vi "SubVI Translate.vi"(8 "error in (no error)":errorcluster, 10 "reentrant VIs":string[](array[string]), 11 "SubVI in":refnum<vi>) -> (0 "error out":errorcluster, 1 "reentrant VIs out":string[](array[string]), 2 "transcripted code":string, 3 "transcriptor cluster":T1)   [LabVIEW 2014]
uses:
  types/LabVIEW Universal Transcriptor Cluster.ctl
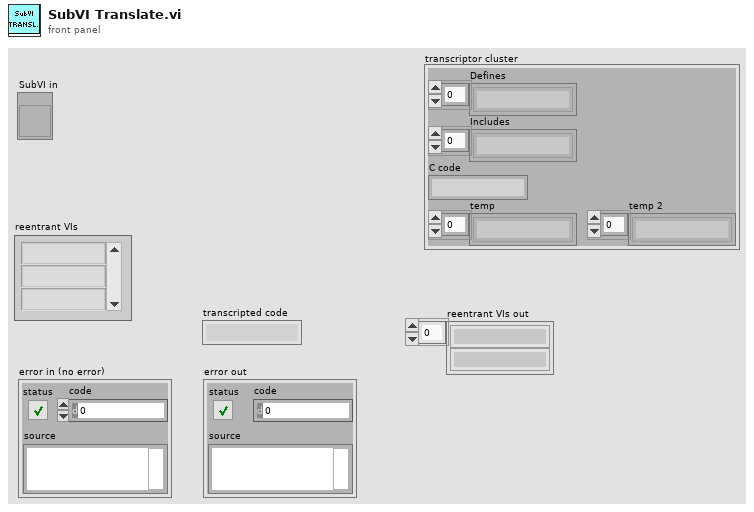
[diagram p1: front panel]
types:
  T1 = typedef "LabVIEW Universal Transcriptor Cluster.ctl" = cluster{"Defines":string[], "Includes":string[], "C code":string, "temp":string[], "temp 2":string[]}
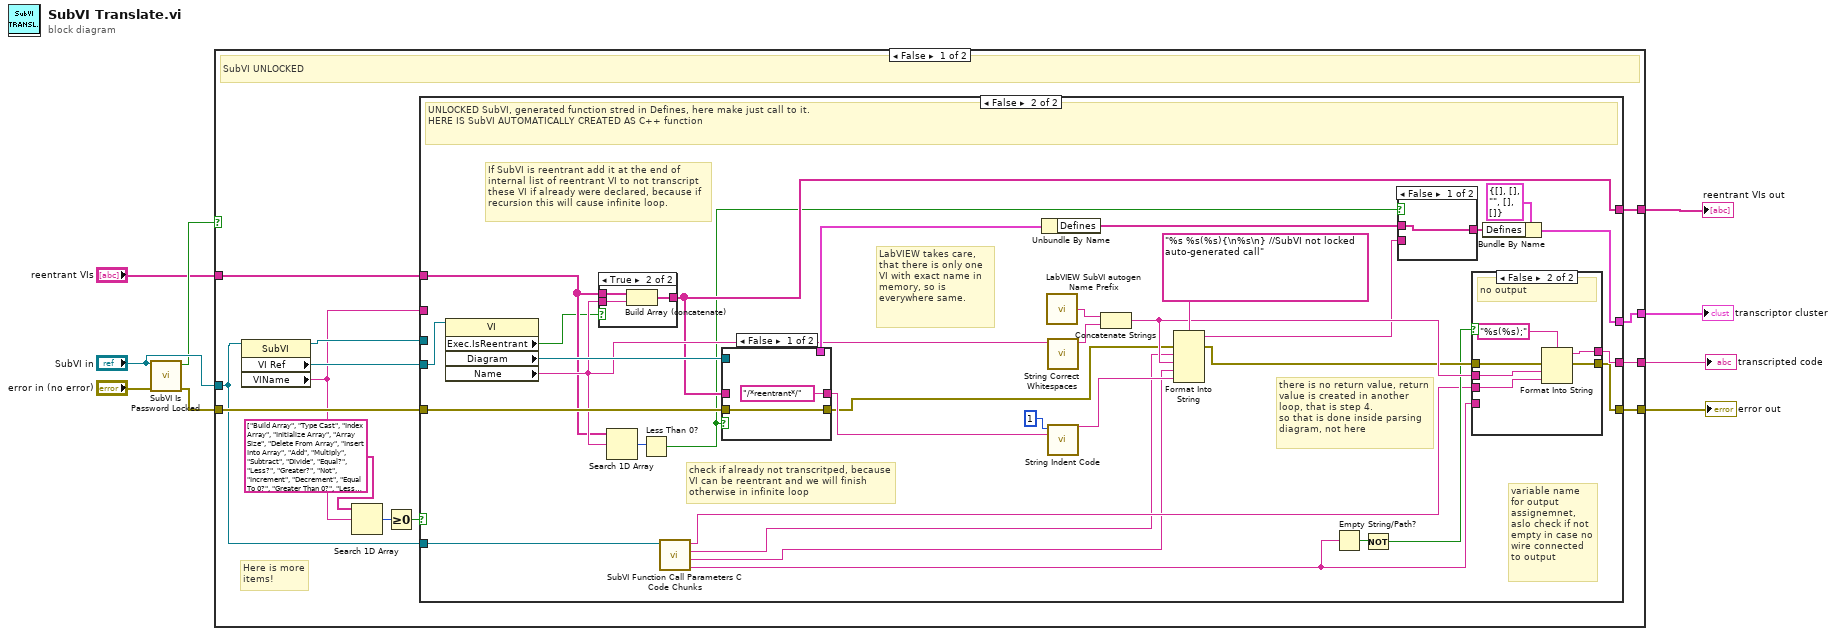
[diagram p0: block diagram]
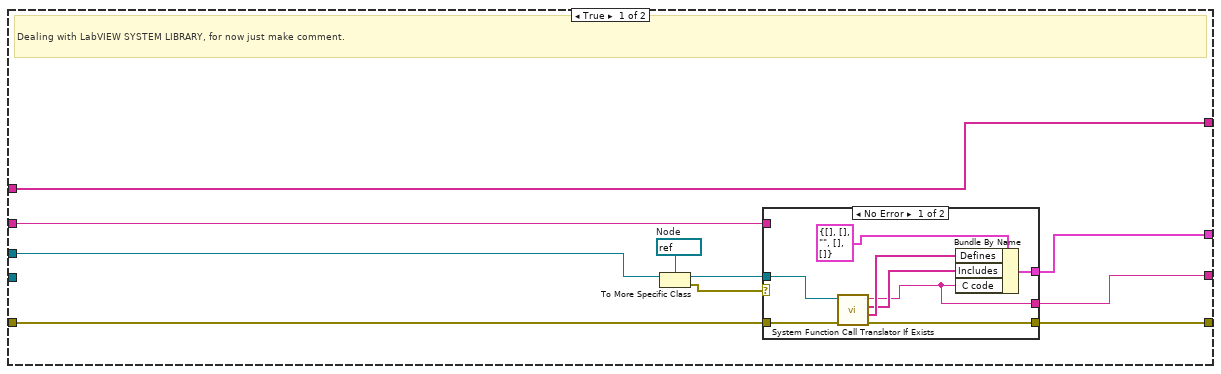
[diagram p2: hidden frame]
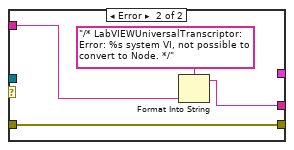
[diagram p3: hidden frame]
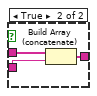
[diagram p4: hidden frame]
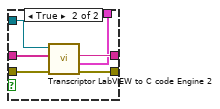
[diagram p6: hidden frame]
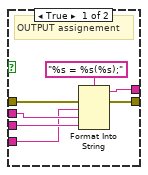
[diagram p7: hidden frame]
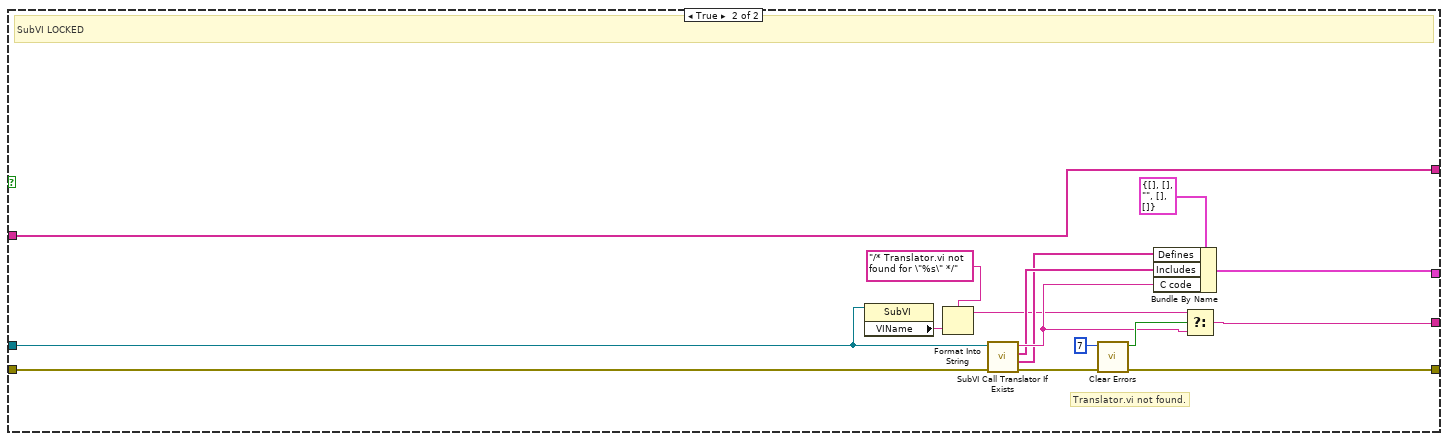
[diagram p8: hidden frame]
diagram:
  n1 = call "SubVI Is Password Locked.vi"("Error In"="error in (no error)", "SubVI ref"="SubVI in") -> ("Error Out"=w8:errorcluster, "isPasswordLocked?"=w5:bool)  [unwired: 8 in]
  n2 = case shown="False" w5 {
    tunnel: "SubVI in" -> [w12 w118]
    tunnel: [w20 w122] -> w7
    tunnel: w8 -> [w22 w121]
    tunnel: [w19 w120] -> w9
    tunnel: [w18 w119] -> w4
    tunnel: "reentrant VIs" -> [w11 w107]
    tunnel: [w10 w107] -> w1
    frame False {
      # "Here is more items!"
      # "SubVI UNLOCKED"
      n3 = property class="SubVI"(reference=w12) -> (reference out=w17:refnum<vi>, "VI Ref"=w21:refnum<vi>, "VIName"=w13:string)  [unwired: 1 in, 1 out]
      n4 = Search 1D Array(1D array=string[] ["Build Array", "Type Cast", "Index Array", "Initialize Array", "Array Size", "Delete From Array", "Insert Into Array", "Add", "Multiply", "Subtract", "Divide", "Equal?", "Less?", "Greater?", "Not", "Increment", "Decrement", "Equal To 0?", "Greater Than 0?", "Less Than 0?", "Greater Or Equal To 0?", "Greater Or Equal?", "Less Or Equal?", "Not Equal?", "Not Equal To 0?", "And", "Or", "Exclusive Or", "To Lower Case", "To Upper Case", "String Length", "String Subset", "Match Pattern", "Decimal String To Number", "Number To Fractional String", "Fract/Exp String To Number", "Number To Decimal String"], element=w13) -> (index of element=w16:i32)  [unwired: 1 in]
      n5 = Greater Or Equal To 0?(x=w16) -> (x >= 0?=w15:bool)
      n6 = case shown="False" w15 {
        tunnel: w22 -> [w30 w52]
        tunnel: w21 -> [_ w64]
        tunnel: [w32 w76] -> w20
        tunnel: [w29 w66] -> w19
        tunnel: w13 -> [w31 _]
        tunnel: [w27 w77] -> w18
        tunnel: w12 -> [_ w62]
        tunnel: w17 -> [w28 _]
        tunnel: w11 -> [w23 w48]
        tunnel: [w23 w47] -> w10
        frame True {
          w26 = refnum<vi> refnum  # Node
          # "Dealing with LabVIEW SYSTEM LIBRARY, for now just make comment."
          n7 = To More Specific Class(target class=w26, reference=w28) -> (specific class reference=w25:refnum<vi>, error out=w24:errorcluster)  [unwired: 1 in]
          n8 = case shown="No Error" w24 {
            tunnel: [w40 w44] -> w29
            tunnel: w25 -> [w39 _]
            tunnel: [w36 _] -> w27
            tunnel: [w35 w41] -> w32
            tunnel: w30 -> [w34 w44]
            tunnel: w31 -> [_ w42]
            frame No Error {
              n9 = call "System Function Call Translator If Exists.vi"("Error In"=w34, "Node Refnum"=w39) -> ("Error Out"=w40:errorcluster, "Defines"=w38:string[], "Includes"=w37:string[], "Replaced Code"=w35:string)  [unwired: 6 in]
              n10 = Bundle By Name(cluster=T1 {"Defines"=[], "Includes"=[], "C code"="", "temp"=[], "temp 2"=[]} ("input cluster"), "Defines"=w38, "Includes"=w37, "C code"=w35) -> (w36:T1)
            }
            frame Error {
              n11 = Format Into String(format string="/* LabVIEWUniversalTranscriptor: Error: %s system VI, not possible to convert to Node. */" ("Replaced Code"), w42) -> (resulting string=w41:string)  [unwired: 2 in, 1 out]
            }
          }
        }
        frame False {
          # "If SubVI is reentrant add it at the end of internal list of reentrant VI to not transcript these VI if already were declared, because if recursion this will cause infinite loop."
          # "check if already not transcritped, because VI can be reentrant and we will finish otherwise in infinite loop"
          # "variable name for output assignemnet, aslo check if not empty in case no wire connected to output"
          # "there is no return value, return value is created in another loop, that is step 4.\nso that is done inside parsing diagram, not here"
          # "LabVIEW takes care, that there is only one VI with exact name in memory, so is everywhere same."
          # "UNLOCKED SubVI, generated function stred in Defines, here make just call to it.\nHERE IS SubVI AUTOMATICALLY CREATED AS C++ function"
          n12 = property class="VI"(reference=w64) -> ("Exec.IsReentrant"=w46:bool, "Diagram"=w65:refnum<vi>, "Name"=w49:string)  [unwired: 1 in, 2 out]
          n13 = case shown="True" w46 {
            tunnel: w49 -> [_ w85]
            tunnel: w48 -> [w82 w84]
            tunnel: [w82 w83] -> w47
            frame False {
            }
            frame True {
              n14 = Build Array (concatenate)(w84, w85) -> (w83:string[])
            }
          }
          n15 = Search 1D Array(1D array=w48, element=w49) -> (index of element=w51:i32)  [unwired: 1 in]
          n16 = Less Than 0?(x=w51) -> (x < 0?=w45:bool)
          n17 = call "SubVI Function Call Parameters C Code Chunks.vi"("SubVI Refnum"=w62) -> ("SubVI output variable name"=w60:string, "SubVI func. declaration"=w53:string, "return datatype"=w54:string, "SubVI func. call in code"=w55:string)  [unwired: 5 in, 2 out]
          n18 = case shown="False" w45 {
            tunnel: w52 -> [w87 w93]
            tunnel: [w87 w92] -> w50
            tunnel: ["/*reentrant*/" ("transcripted code") w91] -> w74
            tunnel: w65 -> [_ w90]
            tunnel: [_ w89] -> w58
            tunnel: w47 -> [_ w88]
            frame False {
            }
            frame True {
              n19 = call "Transcriptor LabVIEW to C code Engine 2.vi"("Error In"=w93, "List Reentrant VIs"=w88, "Diagram in"=w90) -> ("error out"=w92:errorcluster, "output cluster"=w89:T1, "transcripted code"=w91:string)  [unwired: 4 in, 2 out]
            }
          }
          n20 = Unbundle By Name(w58) -> ("Defines"=w57:string[])
          n21 = call "LabVIEW SubVI autogen Name Prefix.vi"() -> ("datatype prefix"=w72:string)
          n22 = call "String Correct Whitespaces.vi"("String in"=w49) -> ("String out"=w71:string)  [unwired: 10 in]
          n23 = call "String Indent Code.vi"("complete code"=w74, "actual nested level"=1) -> ("indented code"=w63:string)  [unwired: 9 in]
          n24 = Concatenate Strings(w72, w71) -> (w70:string)
          n25 = Format Into String(format string="%s %s(%s){\n%s\n} //SubVI not locked auto-generated call", error in=w50, w54, w70, w53, w63) -> (resulting string=w68:string, error out=w67:errorcluster)  [unwired: 1 in]
          n26 = Empty String/Path?(string/path=w60) -> (empty?=w61:bool)
          n27 = Not(x=w61) -> (.not. x?=w59:bool)
          n28 = case shown="False" w45 {
            tunnel: [w78 w81] -> w69
            tunnel: w68 -> [_ w80]
            tunnel: w57 -> [w78 w79]
            frame False {
            }
            frame True {
              n29 = Build Array (concatenate)(w79, w80) -> (w81:string[])
            }
          }
          n30 = case shown="False" w59 {
            tunnel: [w100 w106] -> w76
            tunnel: w70 -> [w98 w104]
            tunnel: w67 -> [w97 w103]
            tunnel: [w96 w102] -> w66
            tunnel: w55 -> [w95 w101]
            tunnel: w60 -> [w94 _]
            frame True {
              # "OUTPUT assignement"
              n31 = Format Into String(format string="%s = %s(%s);", error in=w97, w94, w98, w95) -> (resulting string=w100:string, error out=w96:errorcluster)  [unwired: 1 in]
            }
            frame False {
              # "no output"
              n32 = Format Into String(format string="%s(%s);", error in=w103, w104, w101) -> (resulting string=w106:string, error out=w102:errorcluster)  [unwired: 1 in]
            }
          }
          n33 = Bundle By Name(cluster=T1 {"Defines"=[], "Includes"=[], "C code"="", "temp"=[], "temp 2"=[]} ("input cluster"), "Defines"=w69) -> (w77:T1)
        }
      }
    }
    frame True {
      # "Translator.vi not found."
      # "SubVI LOCKED"
      n34 = property class="SubVI"(reference=w118) -> ("VIName"=w111:string)  [unwired: 1 in, 2 out]
      n35 = Format Into String(format string="/* Translator.vi not found for \"%s\" */" ("t"), w111) -> (resulting string=w109:string)  [unwired: 2 in, 1 out]
      n36 = call "SubVI Call Translator If Exists.vi"("Error In"=w121, "SubVI Refnum"=w118) -> ("Error Out"=w117:errorcluster, "Defines"=w112:string[], "Includes"=w113:string[], "Replaced Code"=w114:string)  [unwired: 6 in]
      n37 = call <vilib>:"Clear Errors.vi"("error in (no error)"=w117, "specific error code to clear (0: all)"=7) -> ("error out"=w120:errorcluster, "specific error cleared?"=w115:bool)  [unwired: 4 in]
      n38 = Bundle By Name(cluster=T1 {"Defines"=[], "Includes"=[], "C code"="", "temp"=[], "temp 2"=[]} ("input cluster"), "Defines"=w112, "Includes"=w113, "C code"=w114) -> (w119:T1)
      n39 = Select(t=w109, s=w115, f=w114) -> (s? t:f=w122:string)
    }
  }
  "error out" <- w9
  "transcripted code" <- w7
  "transcriptor cluster" <- w4
  "reentrant VIs out" <- w1
